vi "Time delay - ON (SubVI).vi"(7 "Ton":dbl) -> (1 "Output":dbl)   [LabVIEW 2016]
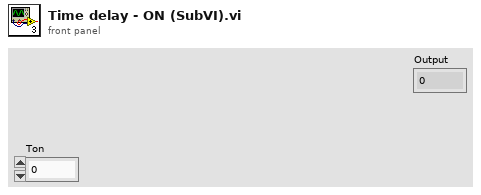
[diagram p1: front panel]
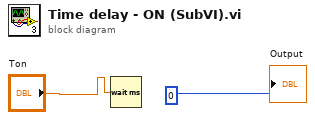
[diagram p0: block diagram]
diagram:
  n1 = Wait (ms)(milliseconds to wait="Ton") -> ()  [unwired: 1 out]
  "Output" <- 0
